vi "CreateSensorSession.vi"(8 "error in (no error)":errorcluster, 11 "RoomAlert in":refnum<class "RoomAlert.lvclass">) -> (0 "error out":errorcluster, 3 "RoomAlert out":refnum<class "RoomAlert.lvclass">)   [LabVIEW 2018, in "SensorPlugins.lvlib" / "RoomAlert.lvclass"]
doc: "Opens a communication link between the application and the RoomAlert Device using the Port number."
uses:
  RoomAlert.lvclass
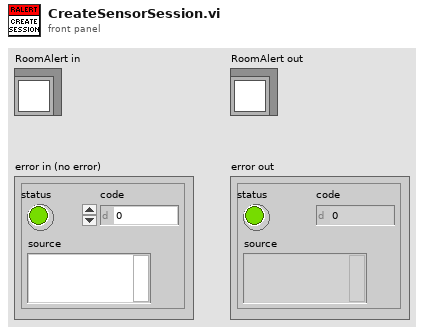
[diagram p1: front panel]
types:
  T1 = typedef "SensorPlugins.lvlib/RoomAlert.lvclass/RoomAlertControls.ctl" = cluster{"Connected?":bool, "IP Address of SNMP Device":string, "Port (161)":u16, "Community Name":string, "Measurements To Read Array":u16[], "Update LightTower?":bool, "LightTower":cluster{"Red":bool, "Amber":bool, "Green":bool, "Audio":bool}, "RoomAlert Model ID":string, "Sensor OID Numbers":string[][], "Sensor Light Tower OID Numbers":string[][]}[]
  T2 = typedef "SensorPlugins.lvlib/RoomAlert.lvclass/CommunicationControls.ctl" = refnum<k16>[]
  T3 = typedef "SensorPlugins.lvlib/RoomAlert.lvclass/MeasurementControls.ctl" = cluster{"Measurement RefreshTime (ms)":u32, "Measurement Name":string, "Timeout(ms)":i32, "Amber Warning Light Configuration":cluster{"Warning Temperture (Degrees C)":dbl, "Temperature Delta (Degrees C/Minute)":dbl, "Time Window (Minutes)":dbl}}
  T4 = cluster{"Connected?":bool, "IP Address of SNMP Device":string, "Port (161)":u16, "Community Name":string, "Measurements To Read Array":u16[], "Update LightTower?":bool, "LightTower":cluster{"Red":bool, "Amber":bool, "Green":bool, "Audio":bool}, "RoomAlert Model ID":string, "Sensor OID Numbers":string[][], "Sensor Light Tower OID Numbers":string[][]}
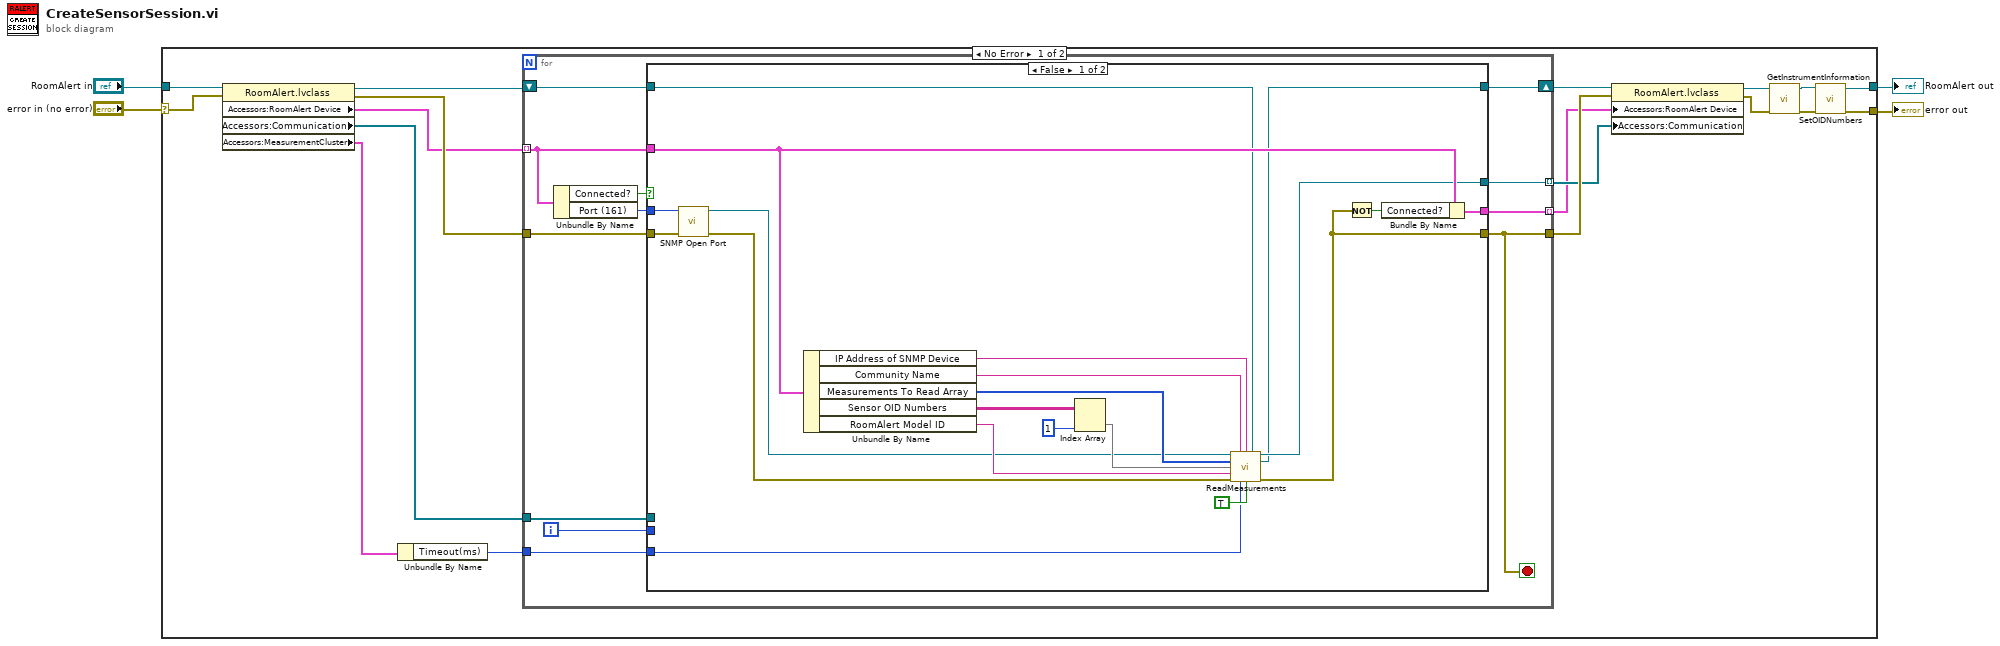
[diagram p0: block diagram]
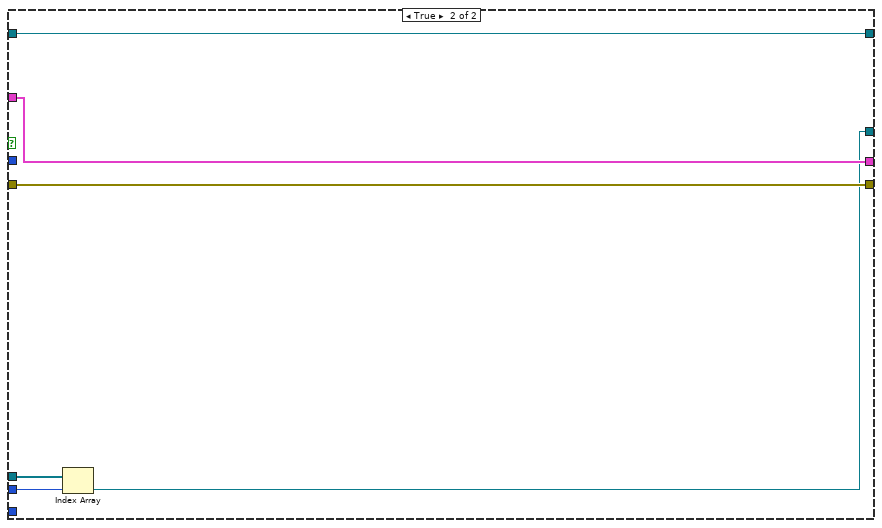
[diagram p2: hidden frame]
diagram:
  n1 = case shown="No Error" "error in (no error)" {
    selector: "error in (no error)" -> [w21 w61]
    tunnel: "RoomAlert in" -> [w22 w62]
    tunnel: [w14 w62] -> w2
    tunnel: [w15 w61] -> w1
    frame No Error {
      n2 = property class="RoomAlert.lvclass"(reference=w22, error in=w21) -> (reference out=w8:refnum<class "RoomAlert.lvclass">, error out=w20:errorcluster, "Accessors:RoomAlert Device"=w9:T1, "Accessors:Communication "=w17:T2, "Accessors:MeasurementCluster"=w6:T3)
      n3 = Unbundle By Name(w6) -> ("Timeout(ms)"=w5:i32)
      n4 = for {
        tunnel: w20 -> [w32]
        tunnel: [w31] -> w19
        tunnel: w9 -> [w34] mode=indexing
        tunnel: [w33] -> w16 mode=indexing
        tunnel: [w26] -> w18 mode=indexing
        tunnel: w17 -> [w27]
        shift-right: [w23] -> w7
        shift-left: w8 -> [w24]
        tunnel: w5 -> [w25]
        i -> [w28]
        stop <- w31 stop-if-true
        n5 = Unbundle By Name(w34) -> ("Connected?"=w29:bool, "Port (161)"=w30:u16)
        n6 = case shown="False" w29 {
          tunnel: w34 -> [w43 w60]
          tunnel: [w54 w60] -> w33
          tunnel: w32 -> [w37 w59]
          tunnel: [w42 w59] -> w31
          tunnel: [w41 w56] -> w26
          tunnel: w30 -> [w52 _]
          tunnel: w28 -> [_ w58]
          tunnel: w27 -> [_ w57]
          tunnel: w25 -> [w40 _]
          tunnel: w24 -> [w38 w55]
          tunnel: [w39 w55] -> w23
          frame False {
            n7 = call "SNMP Open Port.vi"("error in (no error)"=w37, "port"=w52) -> ("error out"=w35:errorcluster, "connection ID"=w36:refnum<k16>)  [unwired: 8 out]
            n8 = Unbundle By Name(w43) -> ("IP Address of SNMP Device"=w50:string, "Community Name"=w51:string, "Measurements To Read Array"=w49:u16[], "Sensor OID Numbers"=w48:string[][], "RoomAlert Model ID"=w44:string)
            n9 = Index Array(array=w48, index (col)=1 ("disabled index (col)")) -> (element=w46:string[])  [unwired: 1 in]
            n10 = call "ReadMeasurements.vi"("UDP Network Connection in"=w36, "Community Name"=w51, "IP Address of SNMP Device"=w50, "RoomAlert in"=w38, "Measurements To Read Array"=w49, "OID Numbers"=w46, "Instrument Model ID"=w44, "error in (no error)"=w35, "Timeout(ms)"=w40, "Filter OID Numbers? (T)"=TRUE) -> ("UDP Network Connection out"=w41:refnum<k16>, "RoomAlert Out"=w39:refnum<class "RoomAlert.lvclass">, "error out"=w42:errorcluster)  [unwired: 2 in, 1 out]
            n11 = Not(x=w42) -> (.not. x?=w53:bool)
            n12 = Bundle By Name(cluster=w43, "Connected?"=w53) -> (w54:T4)
          }
          frame True {
            n13 = Index Array(array=w57, index=w58) -> (element=w56:refnum<k16>)
          }
        }
      }
      n14 = property class="RoomAlert.lvclass"(reference=w7, error in=w19, "Accessors:RoomAlert Device"=w16, "Accessors:Communication "=w18) -> (reference out=w12:refnum<class "RoomAlert.lvclass">, error out=w13:errorcluster)
      n15 = call "GetInstrumentInformation.vi"("error in (no error)"=w13, "RoomAlert in"=w12) -> ("error out"=w11:errorcluster, "RoomAlert out"=w10:refnum<class "RoomAlert.lvclass">)  [unwired: 7 in, 1 out]
      n16 = call "SetOIDNumbers.vi"("error in (no error)"=w11, "RoomAlert in"=w10) -> ("error out"=w15:errorcluster, "RoomAlert out"=w14:refnum<class "RoomAlert.lvclass">)  [unwired: 8 in]
    }
    frame Error {
    }
  }
  "error out" <- w1
  "RoomAlert out" <- w2
